vi "Hang Teleop.vi"(10 "buttons":bool[](array[boolean]), 11 "axis for motor power 2":dbl[](array[numeric])) -> ()   [LabVIEW 2019]
panel:
  in  "axis for motor power 3":dbl[](array[numeric])
  out "motor value":dbl
  in  "axis for motor power":dbl[](array[numeric])
  # "hang (sets motor postiotion to hang/extended)"
  # "activates the ratchet"
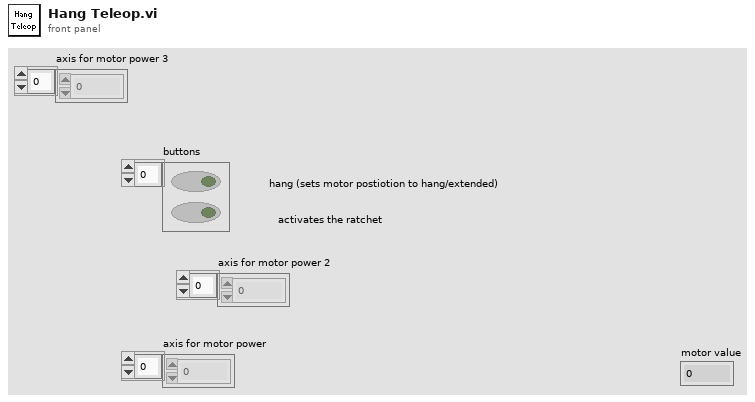
[diagram p1: front panel]
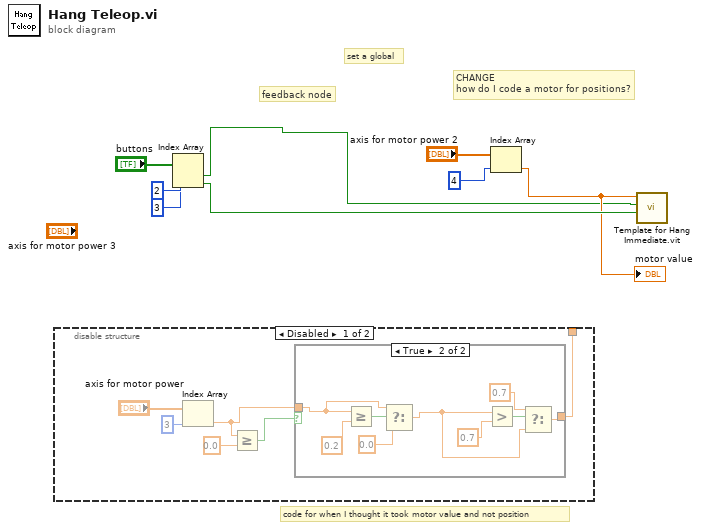
[diagram p0: block diagram]
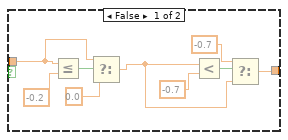
[diagram p2: hidden frame]
diagram:
  # "CHANGE\nhow do I code a motor for positions?"
  # "code for when I thought it took motor value and not position"
  # "set a global"
  # "feedback node"
  n1 = disable-structure shown="Disabled" {
    disable-tunnel: [w9 _] -> _
    frame Disabled {
      n2 = Index Array(array="axis for motor power", index=3) -> (element=w11:dbl)
      n3 = Greater Or Equal?(x=w11, y=0.0) -> (x >= y?=w12:bool)
      n4 = case shown="True" w12 {
        tunnel: w11 -> [w20 w26]
        tunnel: [w15 w24] -> w9
        frame False {
          n5 = Less Or Equal?(x=w20, y=-0.2) -> (x <= y?=w23:bool)
          n6 = Select(t=w20, s=w23, f=0.0) -> (s? t:f=w16:dbl)
          n7 = Less?(x=w16, y=-0.7) -> (x < y?=w18:bool)
          n8 = Select(t=-0.7, s=w18, f=w16) -> (s? t:f=w15:dbl)
        }
        frame True {
          n9 = Greater Or Equal?(x=w26, y=0.2) -> (x >= y?=w32:bool)
          n10 = Select(t=w26, s=w32, f=0.0) -> (s? t:f=w25:dbl)
          n11 = Greater?(x=w25, y=0.7) -> (0:w28:bool)
          n12 = Select(t=0.7, s=w28, f=w25) -> (s? t:f=w24:dbl)
        }
      }
    }
    frame Enabled {
    }
  }
  n13 = Index Array(array="buttons", index #1=2 ("index"), index #2=3 ("index")) -> (element #1=w1:bool, element #2=w7:bool)
  n14 = Index Array(array="axis for motor power 2", index=4) -> (element=w4:dbl)
  "motor value" <- w4
  n15 = call "Template for Hang Immediate.vit"("Ratchet"=w7, "Activation?"=w1, "Motor power"=w4) -> ()  [unwired: 8 in, 1 out]
